vi "Set TreeView.vi"(8 "error in":errorcluster, 10 "Engine":string, 11 "HW Engine in":refnum<class "HW Engine.lvclass">) -> (0 "error out":errorcluster, 2 "Tree DataSet":T1(array[cluster]), 3 "HW Engine out":refnum<class "HW Engine.lvclass">)   [LabVIEW 2025, in "HW Engine.lvlib" / "HW Engine.lvclass"]
uses:
  HW Engine.lvclass
  C:/Users/Public/Documents/Sandia National Labs/TSS Plugin/CEF.lvlibp/Node/CEF_Node.lvclass
  Users/Public/Documents/Sandia National Labs/TSS Plugin/Abstract Engine.lvlibp/Abstract Engine/Abstract Engine.lvclass
  Users/Public/Documents/Sandia National Labs/TSS Plugin/Abstract Engine.lvlibp/Abstract Instrument/Abstract Instrument.lvclass
  Users/Public/Documents/Sandia National Labs/TSS Plugin/CEF.lvlibp/Node/ReadChildren.vi
  Users/Public/Documents/Sandia National Labs/TSS Plugin/Abstract Engine.lvlibp/Abstract Engine/Read Engine Cluster.vi
  Users/Public/Documents/Sandia National Labs/TSS Plugin/Abstract Engine.lvlibp/Abstract Engine/Write Engine Cluster.vi
  Users/Public/Documents/Sandia National Labs/TSS Plugin/CEF.lvlibp/Node/CEF_Node.lvclass
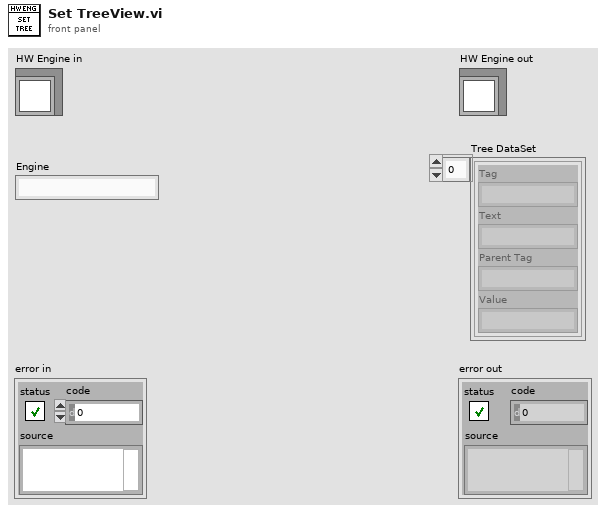
[diagram p1: front panel]
types:
  T1 = cluster{"Tag":string, "Text":string, "Parent Tag":string, "Value":string}[]
  T2 = typedef "Abstract Engine.lvlibp/Abstract Engine.lvclass/Engine Cluster.ctl" = cluster{"IP Address":string, "Type":string, "Initialized":bool, "InstrumentMap":map{string, cluster{"Initialized":bool, "Channels":T3[]}}}
  T3 = typedef "Abstract Engine.lvlibp/Abstract Instrument.lvclass/Channel.ctl" = cluster{"Alias":string, "DataType":enum16{"Anaolg Input", "Waveform"}, "Unit":enum16{"---", "V", "A", "Ohm", "Hz", "uF", "degC", "deg"}, "Upper limit":dbl, "Lower limit":dbl, "Measurement":variant}
  T4 = map{string, cluster{"Initialized":bool, "Channels":T3[]}}
  T5 = cluster{"IP Address":string, "IP Address":string, string, string}
  T6 = cluster{string, "Type":string, "IP Address":string, string}
  T7 = cluster{string, "Instrument":string, string, string}
  T8 = cluster{"IP Address":string, "Alias":string, "IP Address":string, string}[]
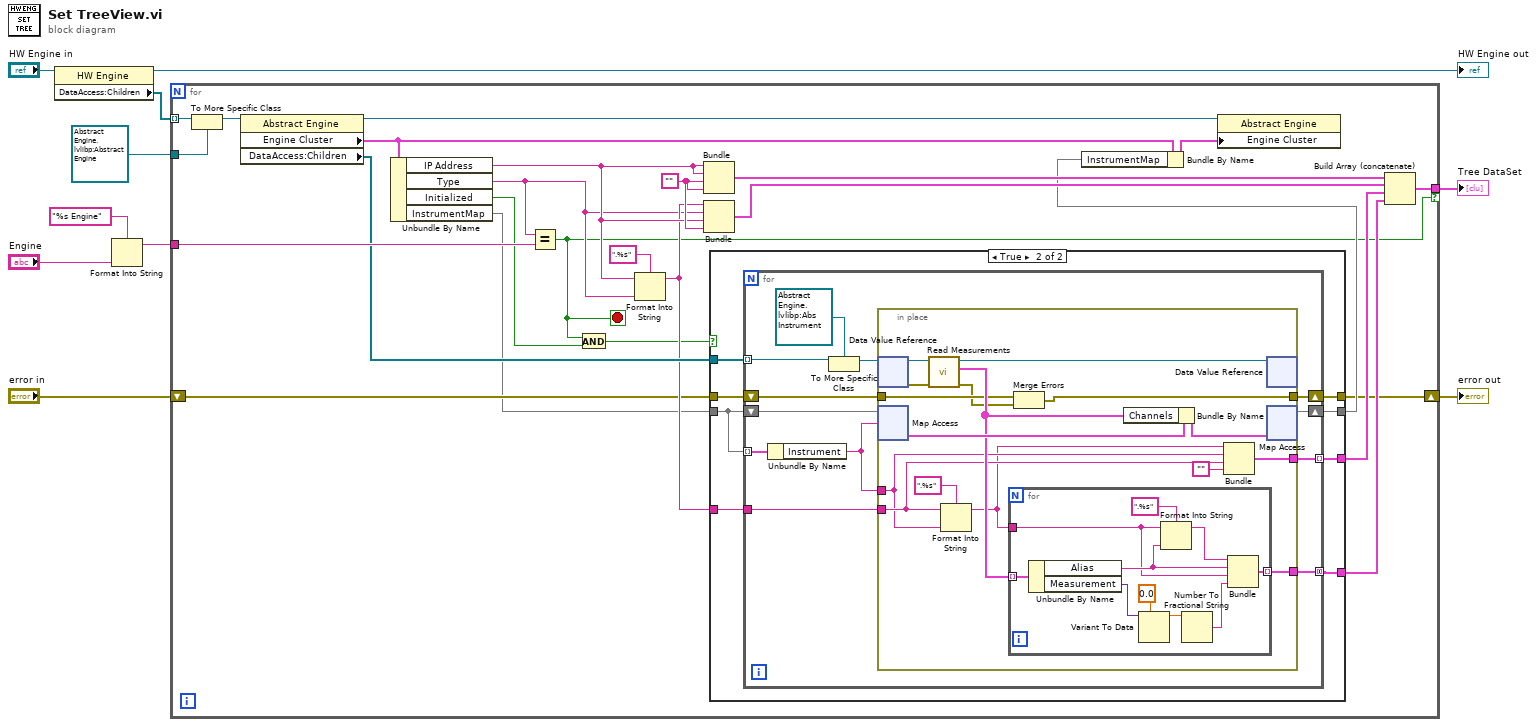
[diagram p0: block diagram]
diagram:
  n1 = property class="HW Engine"(reference="HW Engine in") -> (reference out=→"HW Engine out":refnum<class "HW Engine.lvclass">, "DataAccess:Children"=w5:refnum<data-value>[])  [unwired: 1 in, 1 out]
  n2 = Format Into String(format string="%s Engine", "Engine") -> (resulting string=w6:string)  [unwired: 2 in, 1 out]
  n3 = for {
    tunnel: w6 -> [w33]
    tunnel: w5 -> [w35] mode=indexing
    tunnel: [w26] -> w4 if=w16
    tunnel: refnum<data-value> refnum ("data value reference") -> [w17]
    shift-right: [w12] -> w1
    shift-left: "error in" -> [w13]
    stop <- w16 stop-if-true
    w27 = ""
    n4 = To More Specific Class(target class=w17, reference=w35) -> (specific class reference=w34:refnum<data-value>)  [unwired: 1 in, 1 out]
    n5 = property class="Abstract Engine"(reference=w34) -> (reference out=w32:refnum<data-value>, "Engine Cluster"=w31:T2, "DataAccess:Children"=w23:refnum<data-value>[])  [unwired: 1 in, 1 out]
    n6 = Unbundle By Name(w31) -> ("IP Address"=w24:string, "Type"=w19:string, "Initialized"=w15:bool, "InstrumentMap"=w11:T4)
    n7 = Equal?(x=w19, y=w33) -> (x = y?=w16:bool)
    n8 = And(x=w16, y=w15) -> (x .and. y?=w14:bool)
    n9 = Format Into String(format string=".%s", initial string=w24, w19) -> (resulting string=w22:string)  [unwired: 1 in, 1 out]
    n10 = Bundle("IP Address"=w24, "IP Address"=w24, w27, w27) -> (w29:T5)  [unwired: 1 in]
    n11 = Bundle(w22, "Type"=w19, "IP Address"=w24, w27) -> (w30:T6)  [unwired: 1 in]
    n12 = case shown="True" w14 {
      tunnel: w11 -> [w37 w45]
      tunnel: w23 -> [_ w44]
      tunnel: [w37 w40] -> w18
      tunnel: w22 -> [_ w43]
      tunnel: [_ w42] -> w21
      tunnel: [_ w41] -> w20
      tunnel: w13 -> [w36 w39]
      tunnel: [w36 w38] -> w12
      frame False {
      }
      frame True {
        n13 = for {
          shift-right: [w52] -> w40
          shift-left: w45 -> [w57]
          tunnel: w45 -> [w56] mode=indexing
          tunnel: w44 -> [w54] mode=indexing
          tunnel: w43 -> [w51]
          tunnel: [w49] -> w42 mode=indexing
          tunnel: [w48] -> w41 mode=concatenating
          shift-right: [w47] -> w38
          shift-left: w39 -> [w46]
          n14 = Unbundle By Name(w56) -> ("Instrument"=w50:string)
          n15 = To More Specific Class(target class=refnum<data-value> refnum ("data value reference"), reference=w54) -> (specific class reference=w53:refnum<data-value>)  [unwired: 1 in, 1 out]
          n16 = in-place {
            in-place-border: w51 -> [w66]
            in-place-border: w50 -> [w65]
            in-place-border: [w63] -> w49
            in-place-border: [w62] -> w48
            in-place-border: [w59] -> w47
            in-place-border: w46 -> [w60]
            n17 = in-place-dvr #1(w53) -> (w71:refnum<class "Abstract Instrument.lvclass">, w61:errorcluster)
            n18 = in-place-map #2(w57, w50) -> (w73:cluster{"Initialized":bool, "Channels":T3[]})  [unwired: 1 in, 1 out]
            n19 = call-dynamic "Read Measurements.vi"("error in (no error)"=w61, "Abs Instrument in"=w71) -> ("error out"=w58:errorcluster, "Measurements"=w69:T3[], "Abs Instrument out"=w70:refnum<class "Abstract Instrument.lvclass">)  [unwired: 7 in]
            n20 = Format Into String(format string=".%s", initial string=w66, w65) -> (resulting string=w64:string)  [unwired: 1 in, 1 out]
            n21 = for {
              tunnel: w69 -> [w83] mode=indexing
              tunnel: w64 -> [w79]
              tunnel: [w78] -> w62 mode=indexing
              n22 = Unbundle By Name(w83) -> ("Alias"=w80:string, "Measurement"=w77:variant)
              n23 = Variant To Data(type=0.0, Variant=w77) -> (data=w75:dbl)  [unwired: 1 in, 1 out]
              n24 = Format Into String(format string=".%s", initial string=w79, w80) -> (resulting string=w81:string)  [unwired: 1 in, 1 out]
              n25 = Number To Fractional String(number=w75) -> (F-format string=w74:string)  [unwired: 3 in]
              n26 = Bundle(w81, "Alias"=w80, w79, w74) -> (w78:cluster{string, "Alias":string, string, string})  [unwired: 1 in]
            }
            n27 = Merge Errors(w60, w58) -> (w59:errorcluster)
            n28 = Bundle By Name(cluster=w73, "Channels"=w69) -> (w72:cluster{"Initialized":bool, "Channels":T3[]})
            n29 = Bundle(w64, "Instrument"=w65, w66, "") -> (w63:T7)  [unwired: 1 in]
            n30 = in-place-dvr #1(w70) -> ()  [unwired: 2 out]
            n31 = in-place-map #2(w72) -> (w52:T4)  [unwired: 1 in, 2 out]
          }
        }
      }
    }
    n32 = Bundle By Name(cluster=w31, "InstrumentMap"=w18) -> (w25:T2)
    n33 = property class="Abstract Engine"(reference=w32, "Engine Cluster"=w25) -> ()  [unwired: 1 in, 2 out]
    n34 = Build Array (concatenate)(w29, w30, w21, w20) -> (w26:T8)
  }
  "error out" <- w1
  "Tree DataSet" <- w4
